vi "Cell Weight.vi"(10 "Serial Number":string="1234", 11 "Part Number":string="B0CG1KL3RC") -> (3 "Cell Weight (grams)":dbl=45.0)   [LabVIEW 2024]
panel:
  in  "Cell Weight (grams) 2":dbl=45.0
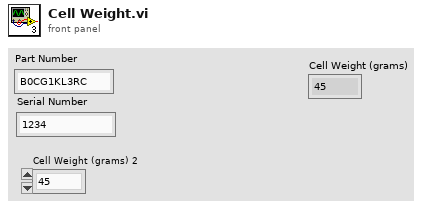
[diagram p1: front panel]
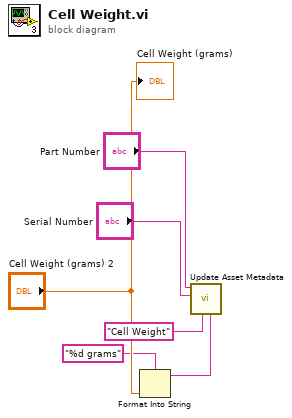
[diagram p0: block diagram]
diagram:
  n1 = Format Into String(format string="%d grams", "Cell Weight (grams) 2") -> (resulting string=w1:string)  [unwired: 2 in, 1 out]
  n2 = call "Update Asset Metadata.vi"("Value"=w1, "Property"="Cell Weight", "Serial Number"="Serial Number", "Part Number"="Part Number") -> ()  [unwired: 6 in, 2 out]
  "Cell Weight (grams)" <- "Cell Weight (grams) 2"
